vi "Execute.vi"(8 "error in (no error)":errorcluster, 10 "Motor in":refnum<class "Motor.lvclass">, 11 "Action in":refnum<class "Action.lvclass">) -> (0 "error out":errorcluster, 1 "Status message":string, 2 "Motor out":refnum<class "Motor.lvclass">, 3 "Action out":refnum<class "Action.lvclass">)   [LabVIEW 2013, in "PowderDeposition.lvlib" / "Action.lvclass"]
uses:
  Action.lvclass
  Motor/Motor.lvclass
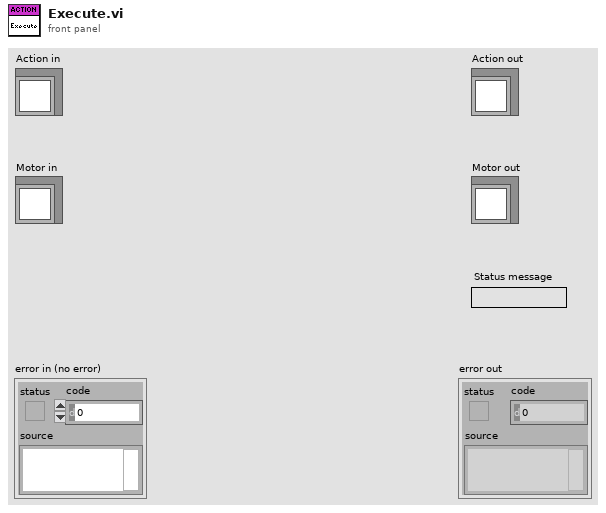
[diagram p1: front panel]
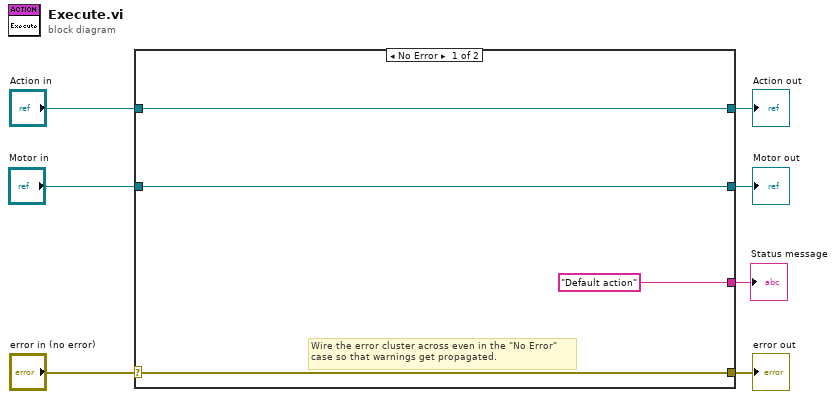
[diagram p0: block diagram]
diagram:
  n1 = case shown="No Error" "error in (no error)" {
    selector: "error in (no error)" -> [w10 w14]
    tunnel: [w10 w14] -> w6
    tunnel: [w11 w13] -> w4
    tunnel: "Action in" -> [w11 w13]
    tunnel: ["Default action" _] -> w3
    tunnel: "Motor in" -> [w8 w12]
    tunnel: [w8 w12] -> w1
    frame No Error {
      # "Wire the error cluster across even in the \"No Error\"\ncase so that warnings get propagated."
    }
    frame Error {
    }
  }
  "error out" <- w6
  "Action out" <- w4
  "Status message" <- w3
  "Motor out" <- w1
